vi "Save_Sequence_of_Unmoving_Dots_To_Matrix-2.vi"(0 "[IN] Stationary Dots":T1(array[cluster]), 1 "# rows":i32, 2 "# cols":i32, 3 "error IN":errorcluster, 4 "[IN] # Gaps":i32) -> (5 "[OUT] FR-TO-FR dot sequence":dbl[][](array[numeric]), 6 "error OUT":errorcluster)   [LabVIEW 2013]
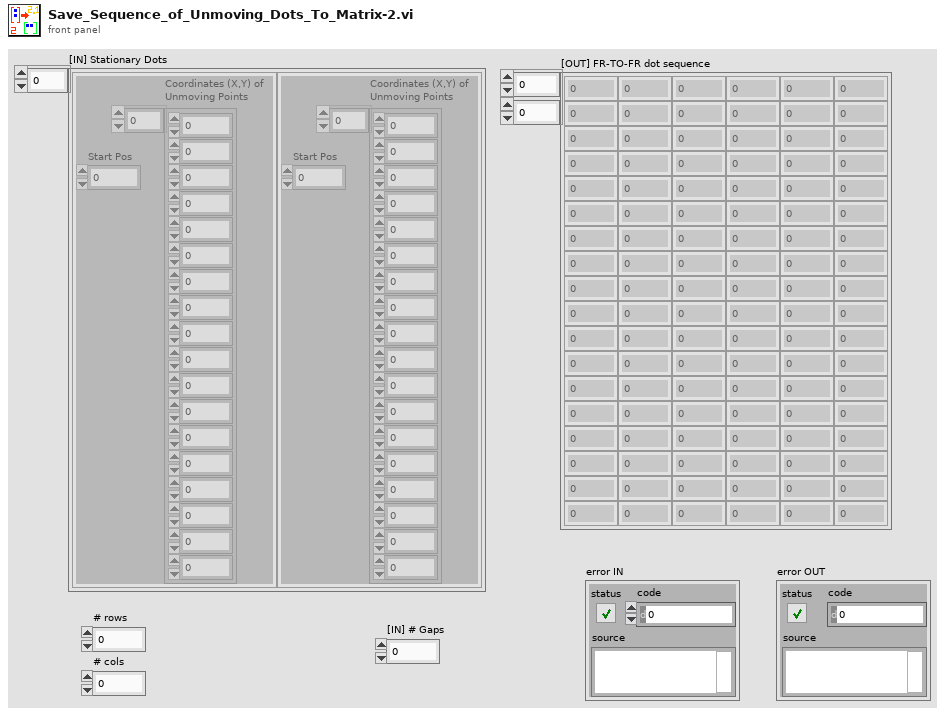
[diagram p1: front panel]
types:
  T1 = cluster{"Coordinates (X,Y) of\nUnmoving Points":dbl[], "Start Pos":i32}[]
  T2 = cluster{"Coordinates (X,Y) of\nUnmoving Points":dbl[], "Start Pos":i32}
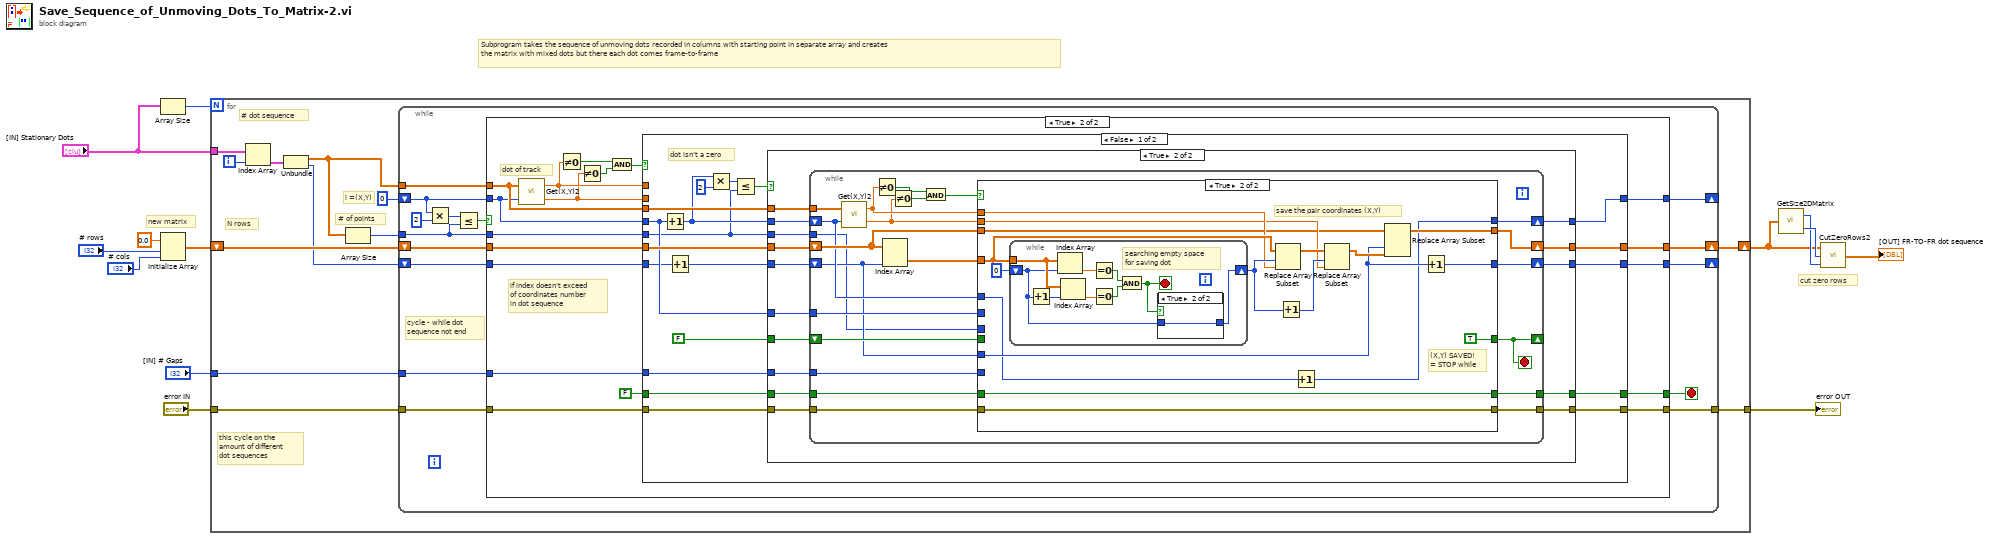
[diagram p0: block diagram]
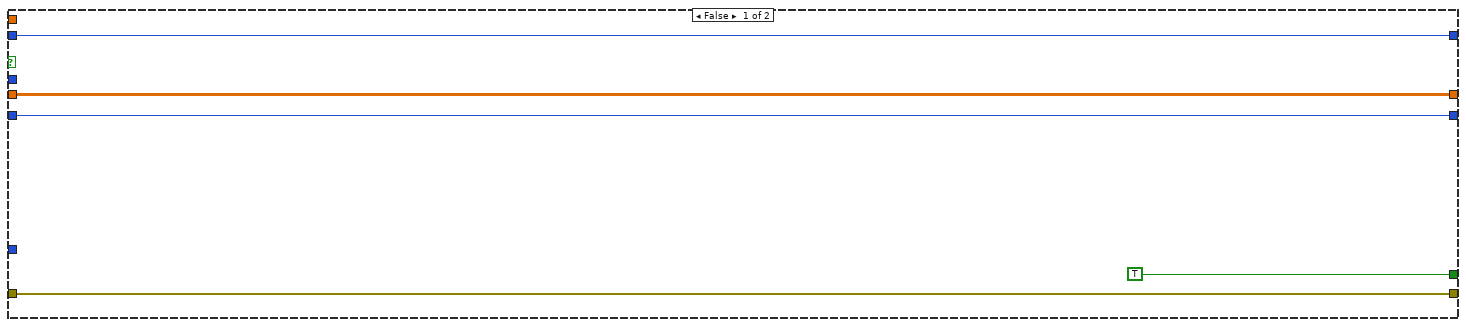
[diagram p2: hidden frame]
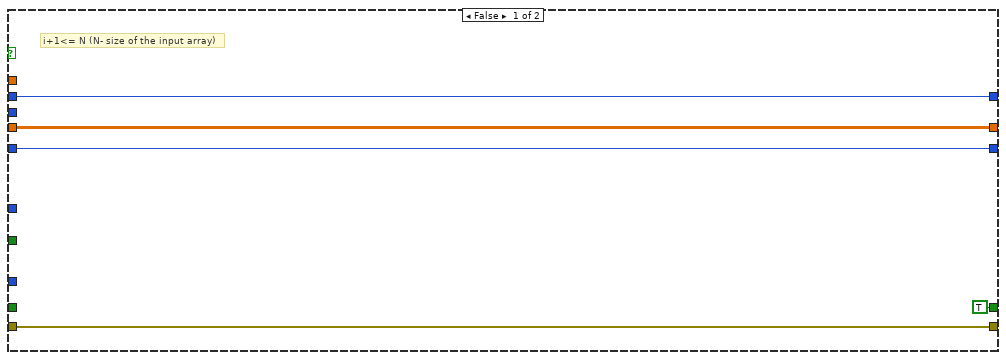
[diagram p3: hidden frame]
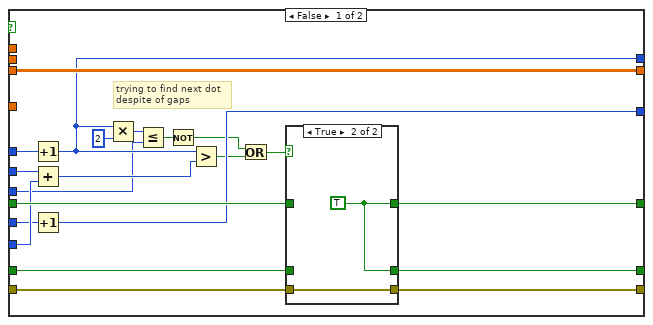
[diagram p4: hidden frame]
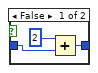
[diagram p6: hidden frame]
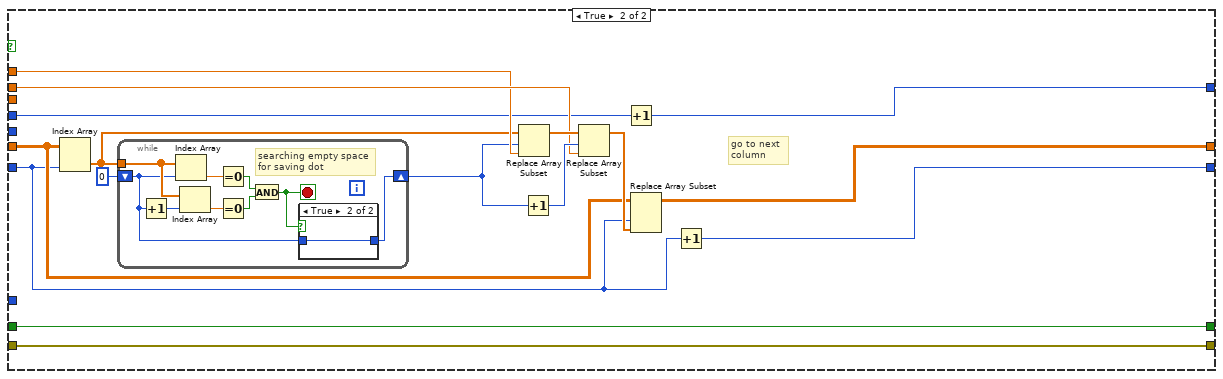
[diagram p7: hidden frame]
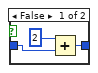
[diagram p8: hidden frame]
diagram:
  # "cut zero rows"
  # "Subprogram takes the sequence of unmoving dots recorded in columns with starting point in separate array and creates \nthe matrix with mixed dots but there each dot comes frame-to-frame"
  # "new matrix"
  n1 = Array Size(array="[IN] Stationary Dots") -> (size(s)=w2:i32)
  n2 = Initialize Array(0.0 ("element"), "# rows", "# cols") -> (w10:dbl[][])
  n3 = for {
    N: w2 -> [_]
    shift-right: [w24] -> w4
    shift-left: w10 -> [w25]
    tunnel: "[IN] # Gaps" -> [w22]
    tunnel: "error IN" -> [w21]
    tunnel: [w20] -> w5
    tunnel: "[IN] Stationary Dots" -> [w19]
    i -> [w18]
    # "# of points"
    # "i =(X,Y)"
    # "N rows"
    # "this cycle on the \namount of different\ndot sequences"
    # "# dot sequence"
    n4 = Index Array(array=w19, index=w18) -> (element=w17:T2)
    n5 = Unbundle(w17) -> ("Coordinates (X,Y) of\nUnmoving Points"=w15:dbl[], "Start Pos"=w16:i32)
    n6 = Array Size(array=w15) -> (size(s)=w14:i32)
    n7 = while {
      tunnel: w15 -> [w37]
      shift-right: [w39] -> w24
      shift-left: w25 -> [w36]
      shift-right: [w40] -> _
      shift-left: w16 -> [w35]
      shift-right: [w38] -> _
      shift-left: 0 -> [w30]
      tunnel: w22 -> [w34]
      tunnel: w14 -> [w27]
      tunnel: w21 -> [w32]
      tunnel: [w31] -> w20
      stop <- w33 stop-if-true
      # "cycle - while dot\nsequence not end"
      n8 = Multiply(x=w30, y=2) -> (x*y=w28:i32)
      n9 = Less Or Equal?(x=w28, y=w27) -> (x <= y?=w26:bool)
      n10 = case shown="True" w26 {
        tunnel: [w44 w61] -> w40
        tunnel: [w45 w60] -> w39
        tunnel: [w41 w59] -> w38
        tunnel: w37 -> [_ w56]
        tunnel: w30 -> [w41 w55]
        tunnel: w27 -> [_ w54]
        tunnel: w36 -> [w45 w53]
        tunnel: w35 -> [w44 w52]
        tunnel: w34 -> [_ w51]
        tunnel: [TRUE w48] -> w33
        tunnel: w32 -> [w42 w47]
        tunnel: [w42 w46] -> w31
        frame False {
        }
        frame True {
          # "if index doesn't exceed\nof coordinates number\nin dot sequence"
          # "dot of track"
          n11 = call "Get(X,Y)2.vi"("[IN] index of (X,Y)"=w55, "[IN] Array coordi\nnates (X,Y) in Frame"=w56) -> ("[OUT] Y"=w57:dbl, "[OUT] X"=w58:dbl)
          n12 = Not Equal To 0?(x=w58) -> (x != 0?=w63:bool)
          n13 = Not Equal To 0?(x=w57) -> (x != 0?=w62:bool)
          n14 = And(x=w63, y=w62) -> (x .and. y?=w50:bool)
          n15 = case shown="False" w50 {
            tunnel: w53 -> [w80 w185]
            tunnel: [w79 w194] -> w60
            tunnel: w57 -> [_ w192]
            tunnel: w58 -> [_ w191]
            tunnel: [w77 w190] -> w61
            tunnel: w55 -> [w72 w189]
            tunnel: w51 -> [w82 _]
            tunnel: [w78 w188] -> w59
            tunnel: w56 -> [w81 _]
            tunnel: w52 -> [w70 w184]
            tunnel: w54 -> [w65 _]
            tunnel: FALSE -> [w76 w182]
            tunnel: [w75 w182] -> w48
            tunnel: w47 -> [w74 w181]
            tunnel: [w73 w181] -> w46
            frame False {
              # "dot isn't a zero"
              n16 = Increment(x=w72) -> (x+1=w66:i32)
              n17 = Increment(x=w70) -> (x+1=w69:i32)
              n18 = Multiply(x=w66, y=2) -> (x*y=w67:i32)
              n19 = Less Or Equal?(x=w67, y=w65) -> (x <= y?=w64:bool)
              n20 = case shown="True" w64 {
                tunnel: w82 -> [_ w102]
                tunnel: w81 -> [_ w101]
                tunnel: w66 -> [w85 w100]
                tunnel: w80 -> [w83 w99]
                tunnel: w65 -> [_ w98]
                tunnel: [w83 w97] -> w79
                tunnel: [w85 w96] -> w78
                tunnel: [w84 w95] -> w77
                tunnel: w76 -> [_ w94]
                tunnel: [TRUE w93] -> w75
                tunnel: w74 -> [w87 w92]
                tunnel: [w87 w91] -> w73
                tunnel: w72 -> [_ w90]
                tunnel: FALSE -> [_ w89]
                tunnel: w69 -> [w84 w88]
                frame False {
                  # "i+1<= N (N- size of the input array)"
                }
                frame True {
                  n21 = while {
                    shift-right: [w113] -> w96
                    shift-left: w100 -> [w116]
                    tunnel: w102 -> [w114]
                    tunnel: w101 -> [w124]
                    shift-right: [w115] -> w97
                    shift-left: w99 -> [w118]
                    tunnel: w98 -> [w103]
                    shift-right: [w117] -> w95
                    shift-left: w88 -> [w104]
                    tunnel: w94 -> [w112]
                    tunnel: [w111] -> w93
                    tunnel: w92 -> [w110]
                    tunnel: [w109] -> w91
                    tunnel: w90 -> [w108]
                    shift-right: [w107] -> _
                    shift-left: w89 -> [w106]
                    stop <- w107 stop-if-true
                    n22 = call "Get(X,Y)2.vi"("[IN] index of (X,Y)"=w116, "[IN] Array coordi\nnates (X,Y) in Frame"=w124) -> ("[OUT] Y"=w120:dbl, "[OUT] X"=w121:dbl)
                    n23 = Not Equal To 0?(x=w121) -> (x != 0?=w123:bool)
                    n24 = Index Array(array=w118, index (col)=w104) -> (element=w119:dbl[])  [unwired: 1 in]
                    n25 = Not Equal To 0?(x=w120) -> (x != 0?=w122:bool)
                    n26 = And(x=w123, y=w122) -> (x .and. y?=w105:bool)
                    n27 = case shown="True" w105 {
                      tunnel: w121 -> [_ w162]
                      tunnel: w120 -> [_ w161]
                      tunnel: w106 -> [w144 _]
                      tunnel: w119 -> [_ w163]
                      tunnel: w118 -> [w145 w160]
                      tunnel: w104 -> [w135 w158]
                      tunnel: [w134 w157] -> w117
                      tunnel: w116 -> [w138 w155]
                      tunnel: [w145 w156] -> w115
                      tunnel: w114 -> [w136 _]
                      tunnel: [w143 TRUE] -> w107
                      tunnel: [w130 w154] -> w113
                      tunnel: w112 -> [w142 w152]
                      tunnel: [w141 w152] -> w111
                      tunnel: w110 -> [w140 w151]
                      tunnel: [w139 w151] -> w109
                      tunnel: w108 -> [w137 _]
                      tunnel: w103 -> [w129 _]
                      frame False {
                        # "trying to find next dot\ndespite of gaps"
                        n28 = Increment(x=w138) -> (x+1=w130:i32)
                        n29 = Add(x=w137, y=w136) -> (x+y=w133:i32)
                        n30 = Increment(x=w135) -> (x+1=w134:i32)
                        n31 = Multiply(x=w130, y=2) -> (x*y=w131:i32)
                        n32 = Less Or Equal?(x=w131, y=w129) -> (x <= y?=w128:bool)
                        n33 = Not(x=w128) -> (.not. x?=w126:bool)
                        n34 = Greater?(x=w130, y=w133) -> (0:w127:bool)
                        n35 = Or(x=w126, y=w127) -> (x .or. y?=w125:bool)
                        n36 = case shown="True" w125 {
                          tunnel: w144 -> [w148 _]
                          tunnel: [w148 w150] -> w143
                          tunnel: w142 -> [w147 _]
                          tunnel: [w147 w150] -> w141
                          tunnel: w140 -> [w146 w149]
                          tunnel: [w146 w149] -> w139
                          frame False {
                          }
                          frame True {
                            w150 = TRUE
                          }
                        }
                      }
                      frame True {
                        # "(X,Y) SAVED!\n= STOP while"
                        # "save the pair coordinates (X,Y)"
                        n37 = while {
                          tunnel: w163 -> [w174]
                          shift-right: [w168] -> w164
                          shift-left: 0 -> [w169]
                          stop <- w170 stop-if-true
                          # "searching empty space\nfor saving dot"
                          n38 = Increment(x=w169) -> (x+1=w175:i32)
                          n39 = Index Array(array=w174, index=w169) -> (element=w176:dbl)
                          n40 = Index Array(array=w174, index=w175) -> (element=w173:dbl)
                          n41 = Equal To 0?(x=w176) -> (x = 0?=w172:bool)
                          n42 = Equal To 0?(x=w173) -> (x = 0?=w171:bool)
                          n43 = And(x=w172, y=w171) -> (x .and. y?=w170:bool)
                          n44 = case shown="True" w170 {
                            tunnel: w169 -> [w178 w180]
                            tunnel: [w179 w180] -> w168
                            frame False {
                              n45 = Add(x=2, y=w178) -> (x+y=w179:i32)
                            }
                            frame True {
                            }
                          }
                        }
                        n46 = Replace Array Subset(array=w163, new element=w162, index=w164) -> (w166:dbl[])
                        n47 = Increment(x=w164) -> (x+1=w165:i32)
                        n48 = Increment(x=w155) -> (x+1=w154:i32)
                        n49 = Replace Array Subset(array=w166, new element=w161, index=w165) -> (w159:dbl[])
                        n50 = Replace Array Subset(array=w160, new element=w159, index (col)=w158) -> (w156:dbl[][])  [unwired: 1 in]
                        n51 = Increment(x=w158) -> (x+1=w157:i32)
                      }
                    }
                  }
                }
              }
            }
            frame True {
              # "go to next \ncolumn"
              n52 = Index Array(array=w185, index (col)=w184) -> (element=w183:dbl[])  [unwired: 1 in]
              n53 = while {
                tunnel: w183 -> [w203]
                shift-right: [w197] -> w186
                shift-left: 0 -> [w198]
                stop <- w199 stop-if-true
                # "searching empty space\nfor saving dot"
                n54 = Increment(x=w198) -> (x+1=w204:i32)
                n55 = Index Array(array=w203, index=w198) -> (element=w205:dbl)
                n56 = Index Array(array=w203, index=w204) -> (element=w202:dbl)
                n57 = Equal To 0?(x=w205) -> (x = 0?=w201:bool)
                n58 = Equal To 0?(x=w202) -> (x = 0?=w200:bool)
                n59 = And(x=w201, y=w200) -> (x .and. y?=w199:bool)
                n60 = case shown="True" w199 {
                  tunnel: w198 -> [w207 w209]
                  tunnel: [w208 w209] -> w197
                  frame False {
                    n61 = Add(x=2, y=w207) -> (x+y=w208:i32)
                  }
                  frame True {
                  }
                }
              }
              n62 = Replace Array Subset(array=w183, new element=w191, index=w186) -> (w196:dbl[])
              n63 = Increment(x=w186) -> (x+1=w195:i32)
              n64 = Replace Array Subset(array=w196, new element=w192, index=w195) -> (w193:dbl[])
              n65 = Increment(x=w189) -> (x+1=w188:i32)
              n66 = Replace Array Subset(array=w185, new element=w193, index (col)=w184) -> (w194:dbl[][])  [unwired: 1 in]
              n67 = Increment(x=w184) -> (x+1=w190:i32)
            }
          }
        }
      }
    }
  }
  "error OUT" <- w5
  n68 = call "GetSize2DMatrix.vi"("Array IN (2D)"=w4) -> ("# Cols"=w7:i32, "# Rows"=w8:i32)
  n69 = call "CutZeroRows2.vi"("# Cols"=w7, "# Rows"=w8, "Array IN"=w4) -> ("Array OUT"=→"[OUT] FR-TO-FR dot sequence":dbl[][])
